vi "SetInitialDirection.vi"(8 "error in (no error)":errorcluster, 10 "InitialDirection":csg, 11 "reference in":refnum<class "Ball.lvclass">) -> (0 "error out":errorcluster, 3 "reference out":refnum<class "Ball.lvclass">)   [LabVIEW 2010, in "Labricks.lvlib" / "Ball.lvclass"]
doc: "Accesses the initial direction of the ball."
uses:
  Ball.lvclass
  Ball.lvclass/Ball.ctl
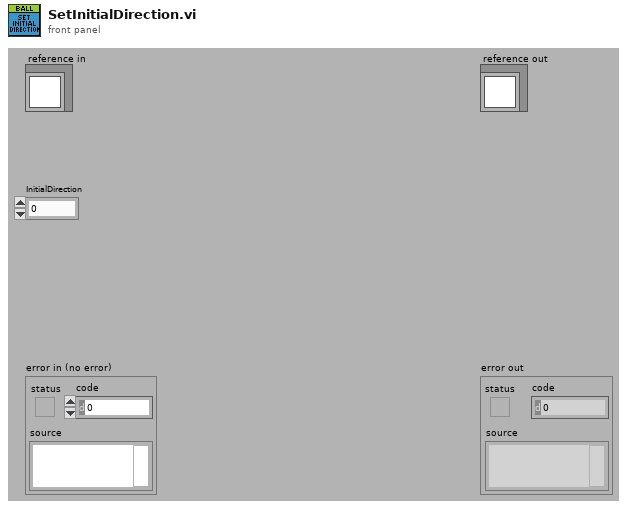
[diagram p1: front panel]
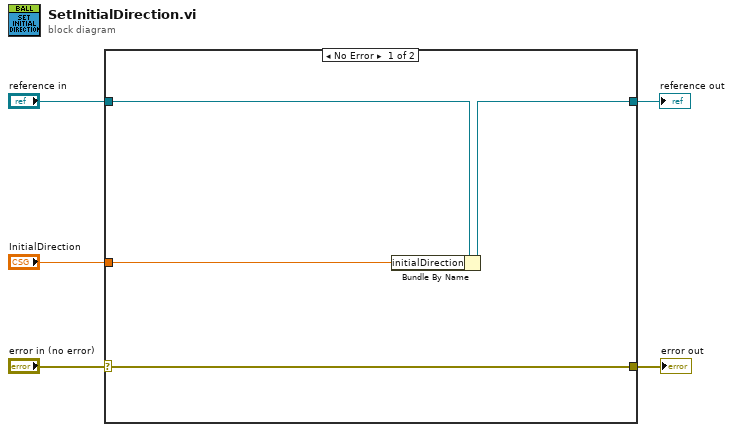
[diagram p0: block diagram]
diagram:
  n1 = case shown="No Error" "error in (no error)" {
    selector: "error in (no error)" -> [w6 w11]
    tunnel: [w6 w11] -> w4
    tunnel: [w8 w10] -> w2
    tunnel: "reference in" -> [w9 w10]
    tunnel: "InitialDirection" -> [w7 _]
    frame No Error {
      n2 = Bundle By Name(cluster=w9, "initialDirection"=w7) -> (w8:refnum<class "Ball.lvclass">)
    }
    frame Error {
    }
  }
  "error out" <- w4
  "reference out" <- w2
